vi "CTRE_CANTalonSRX_ConfigLimitSwitches.vi"(0 "CAN Talon SRX Ref":T1={"DeviceStatus"={"status"=FALSE, "code"=0, "source"=""}, "Type"=enum."PWM", "PWM"={"PWM Channel"=enum."PWM 1", "DeadBand"={"Name"="", "maxPositivePwm"=0, "minPositivePwm"=0, "centerPwm"=0, "maxNegativePwm"=0, "minNegativePwm"=0, "angularRange"=0}}, "CAN"={"Device Number"=0, "SetOutput VI Ref"=variant(enum8{"Percent VBus", "Current", "Speed", "Position", "Voltage"} enum."Percent VBus"), "GetOutput VI Ref"=variant(refnum<k1> refnum), "Enable VI Ref"=variant(dbl 12.0), "Disable VI Ref"=variant(enum8{"Percent VBus", "Speed", "Position", "Slave", "Unchanged / Invalid", "Voltage Compensation", "Current", "Motion Profile"} enum."Percent VBus"), "Data"=variant}, "Invert"=FALSE}, 7 "Forward Limit Switch Normally Open":bool, 9 "Reverse Limit Switch Normally Open":bool, 11 "error in (no error)":errorcluster) -> (4 "CAN Talon SRX Ref":T1={"DeviceStatus"={"status"=FALSE, "code"=0, "source"=""}, "Type"=enum."PWM", "PWM"={"PWM Channel"=enum."PWM 1", "DeadBand"={"Name"="", "maxPositivePwm"=0, "minPositivePwm"=0, "centerPwm"=0, "maxNegativePwm"=0, "minNegativePwm"=0, "angularRange"=0}}, "CAN"={"Device Number"=0, "SetOutput VI Ref"=variant(enum8{"Percent VBus", "Current", "Speed", "Position", "Voltage"} enum."Percent VBus"), "GetOutput VI Ref"=variant(refnum<k1> refnum), "Enable VI Ref"=variant(dbl 12.0), "Disable VI Ref"=variant(enum8{"Percent VBus", "Speed", "Position", "Slave", "Unchanged / Invalid", "Voltage Compensation", "Current", "Motion Profile"} enum."Percent VBus"), "Data"=variant}, "Invert"=FALSE}, 15 "error out":errorcluster)   [LabVIEW 2016]
doc: "Configure how the limit switches are wired. Specify for each switch if it is wired as <b>Normally Open</b> or <b>Normally Closed</b>. You should wire your switched as <b>Normally Closed</b> for fail-safe operation."
uses:
  <vilib>/Rock Robotics/WPI/MotorControl/WPI_MotorControlDeviceRef.ctl
  <vilib>/Rock Robotics/WPI/MotorControl/WPI_MotorControlType.ctl
  <vilib>/Rock Robotics/SystemInterfaces/DIO/FPGA_DIOPWMChannel.ctl
  <vilib>/Rock Robotics/WPI/PWM/WPI_PWMDeadband.ctl
  <vilib>/Rock Robotics/WPI/ThirdParty/CanMotor/CTRLib-LV-TalonSRX/CTRE_CANTalonSRX_Params.ctl
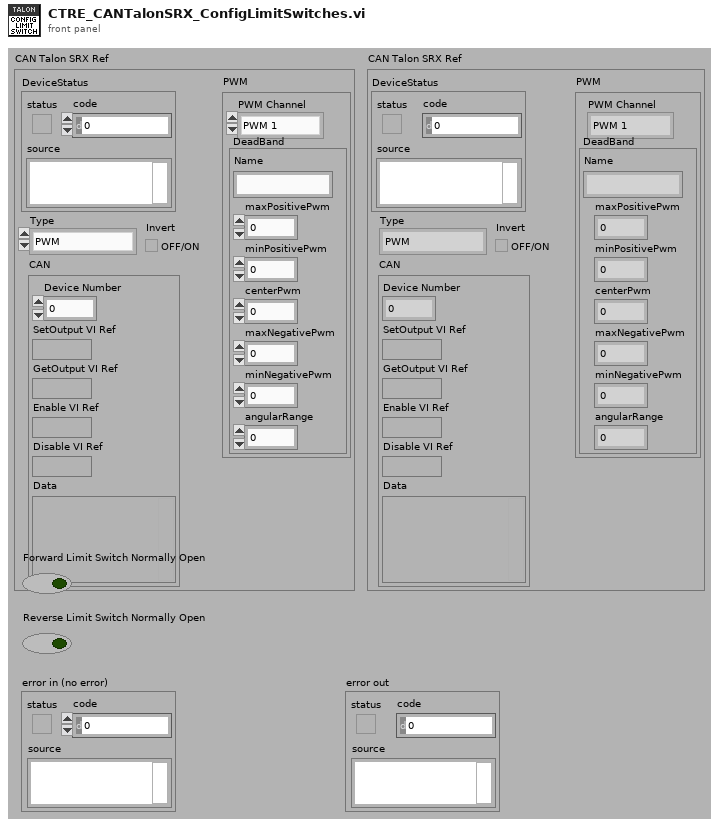
[diagram p1: front panel]
types:
  T1 = typedef "WPI_MotorControlDeviceRef.ctl" = cluster{"DeviceStatus":errorcluster, "Type":T2, "PWM":cluster{"PWM Channel":T3, "DeadBand":T4}, "CAN":cluster{"Device Number":u8, "SetOutput VI Ref":variant, "GetOutput VI Ref":variant, "Enable VI Ref":variant, "Disable VI Ref":variant, "Data":variant}, "Invert":bool}
  T2 = typedef "WPI_MotorControlType.ctl" = enum16{"PWM", "CAN"}
  T3 = typedef "FPGA_DIOPWMChannel.ctl" = enum8{"PWM 0", "PWM 1", "PWM 2", "PWM 3", "PWM 4", "PWM 5", "PWM 6", "PWM 7", "PWM 8", "PWM 9", "PWM MXP 0", "PWM MXP 1", "PWM MXP 2", "PWM MXP 3", "PWM MXP 4", "PWM MXP 5", "PWM MXP 6", "PWM MXP 7", "PWM MXP 8", "PWM MXP 9", "Invalid"}
  T4 = typedef "WPI_PWMDeadband.ctl" = cluster{"Name":string, "maxPositivePwm":i32, "minPositivePwm":i32, "centerPwm":i32, "maxNegativePwm":i32, "minNegativePwm":i32, "angularRange":u16}
  T5 = typedef "CTRE_CANTalonSRX_Params.ctl" = u8
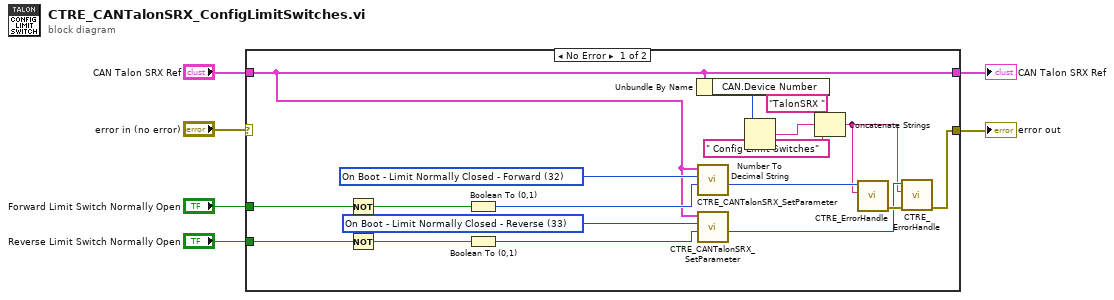
[diagram p0: block diagram]
diagram:
  n1 = case shown="No Error" "error in (no error)" {
    selector: "error in (no error)" -> [_ w26]
    tunnel: [w7 w26] -> w6
    tunnel: [w12 w25] -> w4
    tunnel: "CAN Talon SRX Ref" -> [w12 w25]
    tunnel: "Forward Limit Switch Normally Open" -> [w24 _]
    tunnel: "Reverse Limit Switch Normally Open" -> [w23 _]
    frame No Error {
      w21 = T5 33 items=["Slot 0 - P"=1, "Slot 0 - I"=2, "Slot 0 - D"=3, "Slot 0 - F"=4, "Slot 0 - I Zone"=5, "Slot 0 - Ramp Rate"=6, "Slot 1 - P"=11, "Slot 1 - I"=12, "Slot 1 - D"=13, "Slot 1 - F"=14, "Slot 1 - I Zone"=15, "Slot 1 - Ramp Rate"=16, "Soft Limit - Forward"=21, "Soft Limit - Reverse"=22, "Soft Limit - Forward Enable"=23, "Soft Limit - Reverse Enable"=24, "On Boot - Brake Mode"=31, "On Boot - Limit Normally Closed - Forward"=32, "On Boot - Limit Normally Closed - Reverse"=33, "On Boot - Limit Disabled - Forward"=34, "On Boot - Limit Disabled - Reverse"=35, "Fault - Over Temp"=41, "Fault - Under Voltage"=42, "Fault - Forward Limit"=43, "Fault - Reverse Limit"=44, "Fault - Hardware Failure"=45, "Fault - Forward Soft Limit"=46, "Fault - Reverse Soft Limit"=47, "Sticky Fault - Over Temp"=48, "Sticky Fault - Under Voltage"=49, "Sticky Fault - Forward Limit"=50, "Sticky Fault - Reverse Limit"=51, "Sticky Fault - Forward Soft Limit"=52, "Sticky Fault - Reverse Soft Limit"=53, "Applied Throttle"=61, "Closed-Loop Error"=62, "Select Feedback Device"=63, "Reverse Closed-Loop Output"=64, "Mode Select"=65, "Profile Slot Select"=66, "Ramp Throttle"=67, "Reverse Feedback Sensor"=68, "Limit Switch Enabled"=69, "Limit Switch Closed - Forward"=70, "Limit Switch Closed - Reverse"=71, "Sensor Position"=73, "Sensor Velocity"=74, "Current"=75, "Brake is Enabled"=76, "Encoder Position"=77, "Encoder Velocity"=78, "Encoder Index Rise Events"=79, "Encoder A Pin State"=80, "Encoder B Pin State"=81, "Encoder Index Pin State"=82, "Analog In with Overflow"=83, "Analog In Velocity"=84, "Temperature"=85, "Battery Voltage"=86, "Reset Count"=87, "Reset Flags"=88, "Firmware Version"=89, "Settings Changed"=90] ("Parameter")
      w22 = T5 32 items=["Slot 0 - P"=1, "Slot 0 - I"=2, "Slot 0 - D"=3, "Slot 0 - F"=4, "Slot 0 - I Zone"=5, "Slot 0 - Ramp Rate"=6, "Slot 1 - P"=11, "Slot 1 - I"=12, "Slot 1 - D"=13, "Slot 1 - F"=14, "Slot 1 - I Zone"=15, "Slot 1 - Ramp Rate"=16, "Soft Limit - Forward"=21, "Soft Limit - Reverse"=22, "On Boot - Brake Mode"=31, "On Boot - Limit Normally Closed - Forward"=32, "On Boot - Limit Normally Closed - Reverse"=33, "On Boot - Limit Disabled - Forward"=34, "On Boot - Limit Disabled - Reverse"=35, "Fault - Over Temp"=41, "Fault - Under Voltage"=42, "Fault - Forward Limit"=43, "Fault - Reverse Limit"=44, "Fault - Hardware Failure"=45, "Fault - Forward Soft Limit"=46, "Fault - Reverse Soft Limit"=47, "Sticky Fault - Over Temp"=48, "Sticky Fault - Under Voltage"=49, "Sticky Fault - Forward Limit"=50, "Sticky Fault - Reverse Limit"=51, "Sticky Fault - Forward Soft Limit"=52, "Sticky Fault - Reverse Soft Limit"=53, "Applied Throttle"=61, "Closed-Loop Error"=62, "Select Feedback Device"=63, "Reverse Closed-Loop Output"=64, "Mode Select"=65, "Profile Slot Select"=66, "Ramp Throttle"=67, "Reverse Feedback Sensor"=68, "Limit Switch Enabled"=69, "Limit Switch Closed - Forward"=70, "Limit Switch Closed - Reverse"=71, "Sensor Position"=73, "Sensor Velocity"=74, "Current"=75, "Brake is Enabled"=76, "Encoder Position"=77, "Encoder Velocity"=78, "Encoder Index Rise Events"=79, "Encoder A Pin State"=80, "Encoder B Pin State"=81, "Encoder Index Pin State"=82, "Analog In with Overflow"=83, "Analog In Velocity"=84, "Temperature"=85, "Battery Voltage"=86, "Reset Count"=87, "Reset Flags"=88, "Firmware Version"=89, "Settings Changed"=90] ("Parameter")
      n2 = Not(x=w24) -> (.not. x?=w18:bool)
      n3 = Not(x=w23) -> (.not. x?=w17:bool)
      n4 = Boolean To (0,1)(Boolean=w18) -> (0, 1=w19:i16)
      n5 = Boolean To (0,1)(Boolean=w17) -> (0, 1=w20:i16)
      n6 = Unbundle By Name(w12) -> ("CAN.Device Number"=w13:u8)
      n7 = call <vilib>:"CTRE_CANTalonSRX_SetParameter.vi"("Value"=w19, "Parameter"=w22, "CAN Talon SRX Ref"=w12) -> ("Error Code"=w11:i32)  [unwired: 6 in, 2 out]
      n8 = call <vilib>:"CTRE_CANTalonSRX_SetParameter.vi"("Value"=w20, "Parameter"=w21, "CAN Talon SRX Ref"=w12) -> ("Error Code"=w9:i32)  [unwired: 6 in, 2 out]
      n9 = Number To Decimal String(number=w13) -> (decimal integer string=w15:string)  [unwired: 1 in]
      n10 = Concatenate Strings("TalonSRX " ("string"), w15, " Config Limit Switches" ("string")) -> (w8:string)
      n11 = call <vilib>:"CTRE_ErrorHandle.vi"("origin"=w8, "code"=w11) -> ("error out"=w10:errorcluster)  [unwired: 9 in]
      n12 = call <vilib>:"CTRE_ErrorHandle.vi"("error in"=w10, "origin"=w8, "code"=w9) -> ("error out"=w7:errorcluster)  [unwired: 8 in]
    }
    frame Error {
    }
  }
  "CAN Talon SRX Ref" <- w4
  "error out" <- w6
